vi "Point_in_Triangle2D_Test_PN.vi"(0 "2D Point to Test":dbl[](array[numeric])=[0.0, 0.0], 1 "Triangle2D":T1) -> (2 "Point is in triangle":bool, 3 "w":dbl, 4 "u":dbl, 5 "v":dbl)   [LabVIEW 2010]
uses:
  Triangle2D.ctl
panel:
  in  "1+eps":dbl=1.000000000001 format="%#_16f"
  in  "-eps":dbl=-1e-12 format="%#_16f"
  # "Tests whether the point is inside the triangle or on its edges and returns a boolean result as well as the barycentric coordinate coefficients for carrying out interpolation of vertex values if desired."
  # "Paul Nathan 12/12/09"
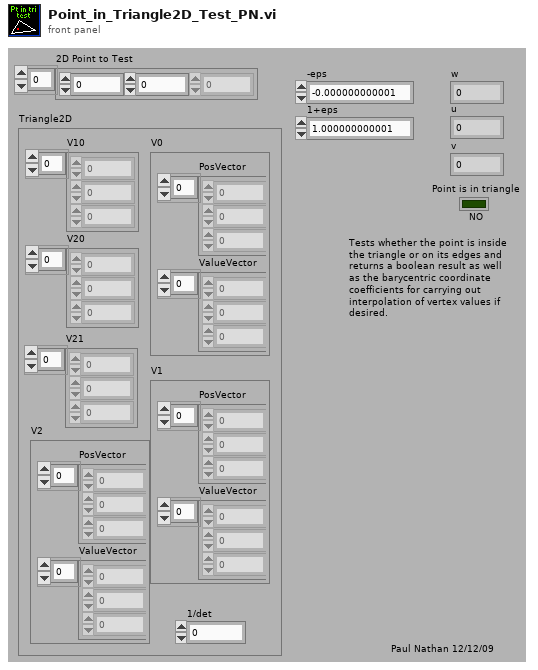
[diagram p1: front panel]
types:
  T1 = typedef "Triangle2D.ctl" = cluster{"V10":dbl[], "V20":dbl[], "1/det":dbl, "V0":cluster{"PosVector":dbl[], "ValueVector":dbl[]}, "V1":cluster{"PosVector":dbl[], "ValueVector":dbl[]}, "V2":cluster{"PosVector":dbl[], "ValueVector":dbl[]}, "V21":dbl[]}
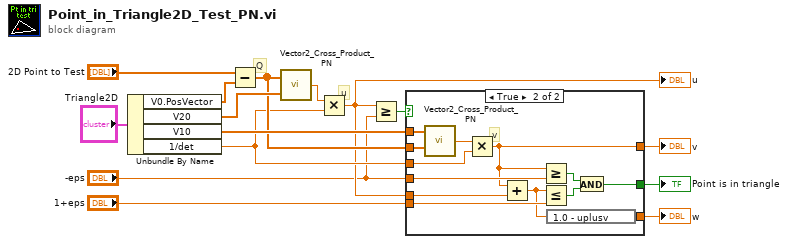
[diagram p0: block diagram]
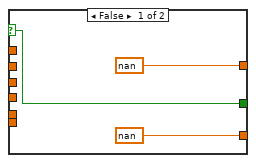
[diagram p2: hidden frame]
diagram:
  # "u"
  # "Q"
  n1 = Unbundle By Name("Triangle2D") -> ("V0.PosVector"=w14:dbl[], "V20"=w13:dbl[], "V10"=w9:dbl[], "1/det"=w7:dbl)
  n2 = Subtract(x="2D Point to Test", y=w14) -> (x-y=w8:dbl[])
  n3 = call "Vector2_Cross_Product_PN.vi"("V (2D)"=w13, "U (2D)"=w8) -> ("U X V (2D)"=w12:dbl)
  n4 = Multiply(x=w12, y=w7) -> (x*y=w2:dbl)
  "u" <- w2
  n5 = Greater Or Equal?(x=w2, y="-eps") -> (x >= y?=w10:bool)
  n6 = case shown="True" w10 {
    selector: w10 -> [w16 _]
    tunnel: w9 -> [_ w30]
    tunnel: w8 -> [_ w29]
    tunnel: w7 -> [_ w28]
    tunnel: "-eps" -> [_ w27]
    tunnel: "1+eps" -> [_ w26]
    tunnel: w2 -> [_ w25]
    tunnel: [nan w23] -> w4
    tunnel: [w16 w20] -> w5
    tunnel: [nan w19] -> w3
    frame False {
    }
    frame True {
      # "v"
      n7 = call "Vector2_Cross_Product_PN.vi"("V (2D)"=w29, "U (2D)"=w30) -> ("U X V (2D)"=w31:dbl)
      n8 = Multiply(x=w31, y=w28) -> (x*y=w19:dbl)
      n9 = Add(x=w19, y=w25) -> (x+y=w24:dbl)
      n10 = Greater Or Equal?(x=w19, y=w27) -> (x >= y?=w21:bool)
      n11 = Less Or Equal?(x=w24, y=w26) -> (x <= y?=w22:bool)
      n12 = expression code="1.0 - uplusv"(w24) -> (w23:dbl)
      n13 = And(x=w21, y=w22) -> (x .and. y?=w20:bool)
    }
  }
  "v" <- w3
  "w" <- w4
  "Point is in triangle" <- w5
